vi "Complex QR Decomposition.vi"(9 "Q option":u16(ring) items=["Full Size Q", "Economy Size Q", "No Q"], 10 "pivot?":bool, 11 "A":T1) -> (0 "error":i32, 1 "P":i32[][](array[numeric]), 2 "R":T1, 3 "Q":T1)   [LabVIEW 2020, in "NI_AALPro.lvlib"]
doc: "Performs the QR decomposition of <B>A</B> with or without column pivoting. Wire data to the <B>A</B> input to determine the polymorphic instance to use or manually select the instance."
uses:
  <vilib>/Analysis/NI_AALPro.lvlib
  <vilib>/Analysis/Matrix/Datatypes/ComplexMatrix.ctl
  <resource>/lvanlys.dll
  <vilib>/Analysis/Matrix/NI_Matrix.lvlib
panel:
  # "QR Decomposition"
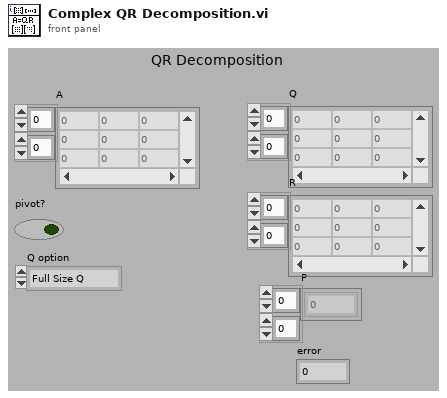
[diagram p1: front panel]
types:
  T1 = typedef "NI_Matrix.lvlib/ComplexMatrix.ctl" = cdb[][]
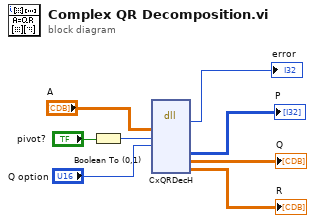
[diagram p0: block diagram]
diagram:
  n1 = Boolean To (0,1)(Boolean="pivot?") -> (0, 1=w4:i16)
  n2 = dll-call lib="e:/builds/penguin/labview/branches/2020/dev/dist/resource/lvanlys.*" fn="CxQRDecH"("A"="A", "pvt"=w4, "qOption"="Q option") -> (→"error":i32, "P"=→"P":i32[][], "Q"=→"Q":T1, "R"=→"R":T1)  [unwired: 9 in, 2 out]
